vi "Query if Galvo or Reso.vi"(8 "error in (no error)":errorcluster) -> (0 "error out":errorcluster, 3 "System Type":enum16{"Galvo", "Reso"}(ring))   [LabVIEW 2012]
doc: "SciScan 1.2 160622"
uses:
  Custom Controls/MAIN Image panel reso tab Control type def.ctl
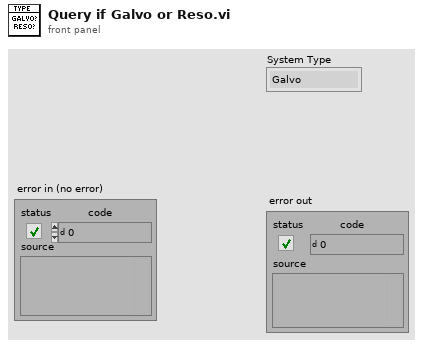
[diagram p1: front panel]
types:
  T1 = typedef "MAIN Image panel reso tab Control type def.ctl" = enum32{"Channel 1", "Channel 2", "Channel 3", "Channel 4", "Channel 5", "all channels", "RGB overlay", "ROI", "arbitrary line scan"}
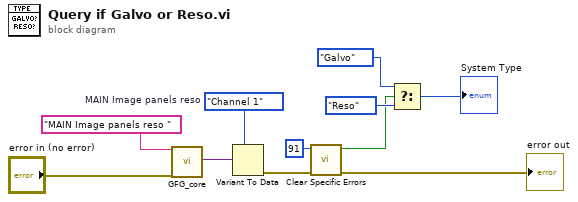
[diagram p0: block diagram]
diagram:
  w10 = MAIN_Image_panel_reso_tab_Control_type_def."Channel 1"  # MAIN Image panels reso
  n1 = call "GFG_core.vi"("Variable Name in"="MAIN Image panels reso ", "error in (no error)"="error in (no error)") -> ("Variant Out"=w9:variant)  [unwired: 11 in, 6 out]
  n2 = Variant To Data(type=w10, Variant=w9) -> (error out=w7:errorcluster)  [unwired: 1 in, 1 out]
  n3 = call "Clear Specific Errors.vi"("Error In"=w7, "Error number In"=91) -> ("Error Out"=→"error out":errorcluster, "Error Cleared?"=w4:bool)  [unwired: 8 in]
  n4 = Select(t=enum16{"Galvo", "Reso"}."Galvo" ("System Type"), s=w4, f=enum16{"Galvo", "Reso"}."Reso") -> (s? t:f=→"System Type":enum16{"Galvo", "Reso"})
